vi "RegWriteExt UnitTest.vi"() -> ()   [LabVIEW 2018]
uses:
  Downloads/MIPI RFFE API/Controls/RFFE Commands Type Def.ctl
  Downloads/MIPI RFFE API/Controls/Write Data Strict Type Def.ctl
  Command/RFFE Command.lvclass
  RegWriteExt/RFFE RegWriteExt Command.lvclass
  C:/Users/semoore/Projects/mipi-rffe-labview-oop/Command/RFFE Command.lvclass
panel:
  out "arrays same size?":bool
  out "data equal?":bool
  out "error in (no error) 2":errorcluster
  in  "error in (no error)":errorcluster
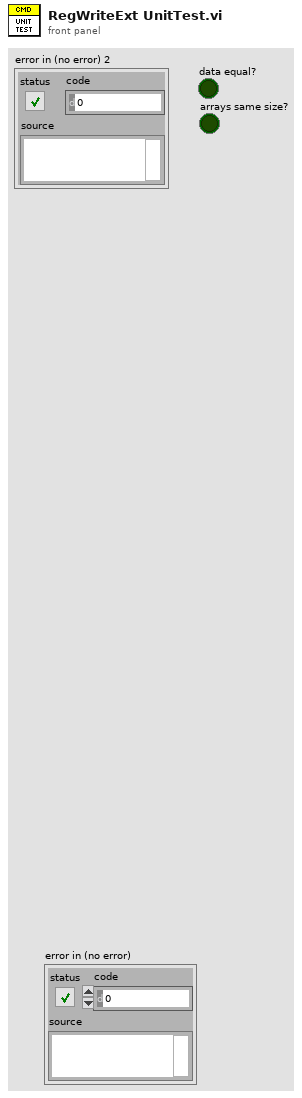
[diagram p1: front panel]
types:
  T1 = typedef "Write Data Strict Type Def.ctl" = cluster{"slave address":u8, "register address":u16, "register data (write)":u8[], "byte count":u8}
  T2 = typedef "RFFE Commands Type Def.ctl" = enum16{"Reg0Write", "RegWrite", "RegRead", "RegReadHR", "RegWriteExt", "RegReadExt", "RegReadExtHR", "RegWriteExtLong", "RegReadExtLong", "RegReadExtLongHR"}
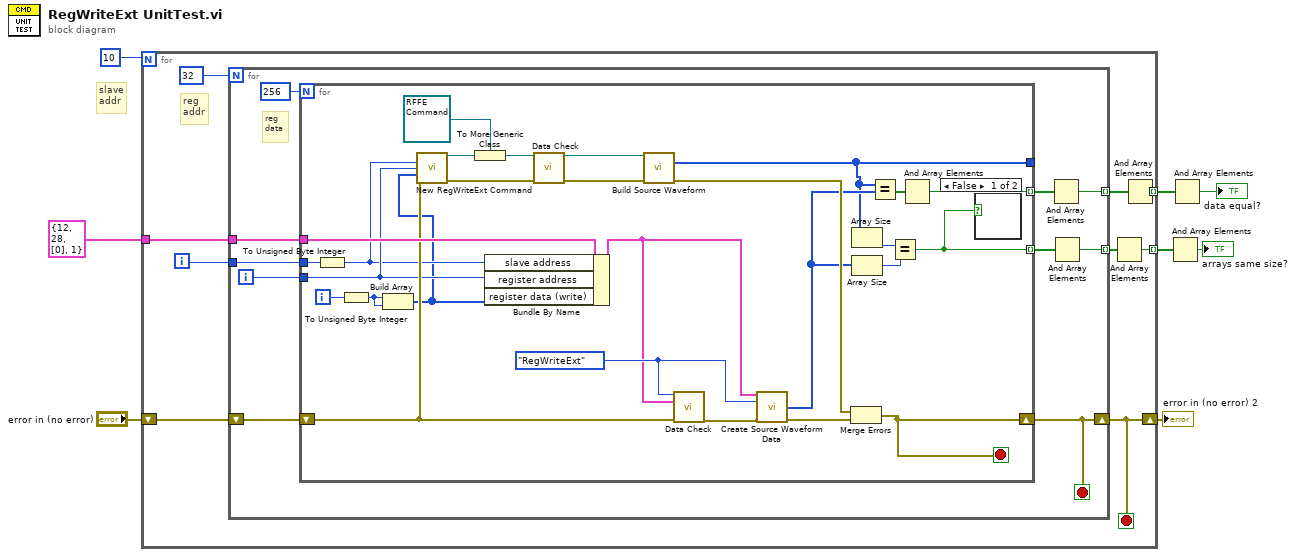
[diagram p0: block diagram]
diagram:
  # "slave\naddr"
  n1 = for {
    N: 10 -> [_]
    tunnel: T1 {"slave address"=12, "register address"=28, "register data (write)"=[0], "byte count"=1} ("Register Data") -> [w16]
    shift-right: [w13] -> w5
    shift-left: "error in (no error)" -> [w17]
    tunnel: [w11] -> w4 mode=indexing
    tunnel: [w9] -> w2 mode=indexing
    i -> [w15]
    stop <- w13 stop-if-true
    # "reg\naddr"
    n2 = for {
      N: 32 -> [_]
      tunnel: w16 -> [w26]
      tunnel: w15 -> [w23]
      shift-right: [w22] -> w13
      shift-left: w17 -> [w27]
      tunnel: [w20] -> w12 mode=indexing
      tunnel: [w18] -> w10 mode=indexing
      i -> [w24]
      stop <- w22 stop-if-true
      # "reg\ndata"
      n3 = for {
        N: 256 -> [_]
        tunnel: w26 -> [w52]
        tunnel: [w38] -> _
        tunnel: w24 -> [w32]
        tunnel: w23 -> [w41]
        shift-right: [w45] -> w22
        shift-left: w27 -> [w42]
        tunnel: [w35] -> w21 mode=indexing
        tunnel: [w28] -> w19 mode=indexing
        i -> [w40]
        stop <- w45 stop-if-true
        w54 = RFFE_Commands_Type_Def."RegWriteExt" ("RFFE command")
        n4 = To Unsigned Byte Integer(number=w41) -> (unsigned 8bit integer=w31:u8)
        n5 = To Unsigned Byte Integer(number=w40) -> (unsigned 8bit integer=w30:u8)
        n6 = Build Array(w30, w30) -> (w29:u8[])
        n7 = call "New RegWriteExt Command.vi"("Slave Address"=w31, "Register Address"=w32, "Register Data"=w29, "error in (no error)"=w42) -> ("RFFE RegWriteExt Command out"=w48:refnum<class "RFFE RegWriteExt Command.lvclass">, "error out"=w49:errorcluster)  [unwired: 10 in]
        n8 = To More Generic Class(target class=refnum<class "RFFE Command.lvclass"> refnum ("RFFE Commands.lvlib:RFFE Command.lvclass"), reference=w48) -> (generic class reference=w34:refnum<class "RFFE Command.lvclass">)
        n9 = Bundle By Name(cluster=w52, "slave address"=w31, "register address"=w32, "register data (write)"=w29) -> (w51:T1)
        n10 = call-dynamic "Data Check.vi"("RFFE Command in"=w34, "error in (no error)"=w49) -> ("RFFE Command out"=w47:refnum<class "RFFE Command.lvclass">, "error out"=w50:errorcluster)  [unwired: 12 in]
        n11 = call-dynamic "Build Source Waveform.vi"("RFFE Command in"=w47, "error in (no error)"=w50) -> ("Source Waveform"=w38:u32[], "error out"=w44:errorcluster)  [unwired: 11 in, 1 out]
        n12 = call "Data Check.vi"("RFFE command"=w54, "Register Data"=w51, "error in"=w42) -> ("error out"=w53:errorcluster)  [unwired: 12 in]
        n13 = call "Create Source Waveform Data.vi"("Register Data"=w51, "RFFE command"=w54, "error in"=w53) -> ("RFFEWrite source waveform data array"=w39:u32[], "error out"=w46:errorcluster)  [unwired: 10 in, 1 out]
        n14 = Merge Errors(w44, w46) -> (w45:errorcluster)
        n15 = Array Size(array=w38) -> (size(s)=w37:i32)
        n16 = Array Size(array=w39) -> (size(s)=w36:i32)
        n17 = Equal?(x=w38, y=w39) -> (x = y?=w43:bool[])
        n18 = Equal?(x=w37, y=w36) -> (x = y?=w28:bool)
        n19 = And Array Elements(Boolean array=w43) -> (logical AND=w35:bool)
        n20 = case shown="False" w28 {
          frame False {
          }
          frame True {
          }
        }
      }
      n21 = And Array Elements(Boolean array=w21) -> (logical AND=w20:bool)
      n22 = And Array Elements(Boolean array=w19) -> (logical AND=w18:bool)
    }
    n23 = And Array Elements(Boolean array=w10) -> (logical AND=w9:bool)
    n24 = And Array Elements(Boolean array=w12) -> (logical AND=w11:bool)
  }
  "error in (no error) 2" <- w5
  n25 = And Array Elements(Boolean array=w2) -> (logical AND=→"arrays same size?":bool)
  n26 = And Array Elements(Boolean array=w4) -> (logical AND=→"data equal?":bool)
